vi "Page_Source_Initialize.vi"(8 "error in (no error)":errorcluster, 9 "ctlReferences":T3, 11 "AB_Build in":refnum<class "AB_Build.lvclass">) -> (0 "error out":errorcluster, 1 "supportedFunctions":T1, 3 "AB_Build out":refnum<class "AB_Build.lvclass">)   [LabVIEW 2020, in "AB_Build.lvclass"]
uses:
  <vilib>/AppBuilder/AB_Classes/Build/AB_Build.lvclass
  <resource>/Framework/Providers/Builds/AppBuilder/AB_UI_Page_Source_Files_References.ctl
  <resource>/Framework/Providers/Builds/AppBuilder/AB_UI_Page_Source_Files_supportedFunctions.ctl
  <vilib>/AppBuilder/AB_Source_Inclusion.ctl
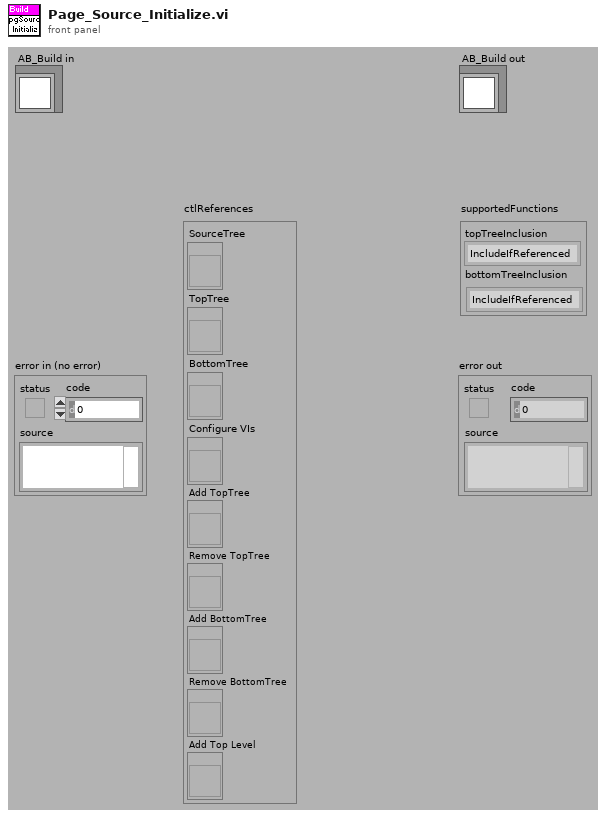
[diagram p1: front panel]
types:
  T1 = typedef "AB_UI_Page_Source_Files_supportedFunctions.ctl" = cluster{"topTreeInclusion":T2, "bottomTreeInclusion":T2}
  T2 = typedef "AB_Source_Inclusion.ctl" = enum16{"IncludeIfReferenced", "Include", "Exclude", "TopLevel"}
  T3 = typedef "AB_UI_Page_Source_Files_References.ctl" = cluster{"SourceTree":refnum<vi>, "TopTree":refnum<vi>, "BottomTree":refnum<vi>, "Configure VIs":refnum<vi>, "Add TopTree":refnum<vi>, "Remove TopTree":refnum<vi>, "Add BottomTree":refnum<vi>, "Remove BottomTree":refnum<vi>, "Add Top Level":refnum<vi>}
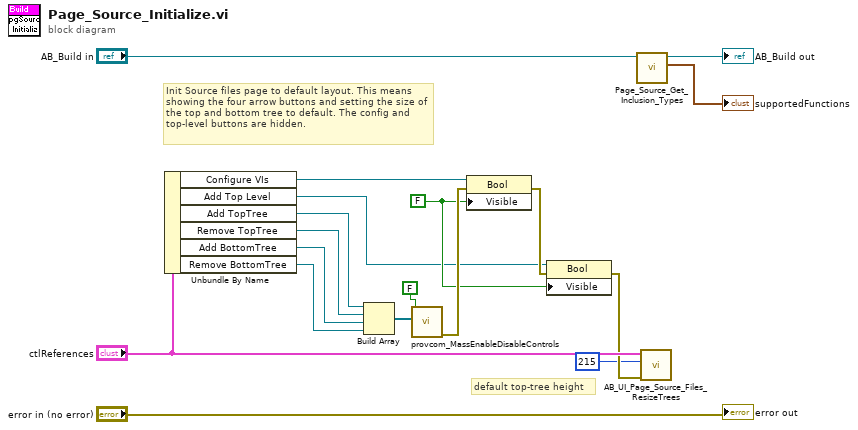
[diagram p0: block diagram]
diagram:
  w11 = FALSE ("Visible")
  # "default top-tree height"
  # "Init Source files page to default layout. This means showing the four arrow buttons and setting the size of the top and bottom tree to default. The config and top-level buttons are hidden."
  n1 = Unbundle By Name("ctlReferences") -> ("Configure VIs"=w8:refnum<vi>, "Add Top Level"=w7:refnum<vi>, "Add TopTree"=w6:refnum<vi>, "Remove TopTree"=w5:refnum<vi>, "Add BottomTree"=w4:refnum<vi>, "Remove BottomTree"=w3:refnum<vi>)
  n2 = Build Array(w6, w5, w4, w3) -> (w9:refnum<vi>[])
  n3 = call <resource>:"provcom_MassEnableDisableControls.vi"("References to alter"=w9, "Enable (TRUE)"=FALSE) -> ("error out"=w12:errorcluster)  [unwired: 1 in, 8 out]
  n4 = property class="Bool"(reference=w8, error in=w12, "Visible"=w11) -> (error out=w13:errorcluster)  [unwired: 1 out]
  n5 = property class="Bool"(reference=w7, error in=w13, "Visible"=w11) -> (error out=w2:errorcluster)  [unwired: 1 out]
  n6 = call-dynamic "Page_Source_Get_Inclusion_Types.vi"("AB_Build in"="AB_Build in") -> ("supportedFunctions"=→"supportedFunctions":T1, "AB_Build out"=→"AB_Build out":refnum<class "AB_Build.lvclass">)  [unwired: 8 in, 1 out]
  n7 = call <resource>:"AB_UI_Page_Source_Files_ResizeTrees.vi"("error in (no error)"=w2, "TopTree height"=215, "ctlReferences"="ctlReferences") -> ()  [unwired: 8 in, 1 out]
  "error out" <- "error in (no error)"
